vi "PDHydra - TVS Test.vi"(8 "error in (no error)":errorcluster, 10 "Message IN":string) -> (0 "error out":errorcluster, 1 "Result (bool)":bool, 2 "Message OUT":string)   [LabVIEW 2022 SP3]
panel:
  in  "bypass":bool
  in  "stop":bool
  out "Instructional Message":string
  in  "OK Button":bool
  out "Actual Breaker AUX state":bool[](array[boolean])
  out "Result (color)":u32(colorbox)
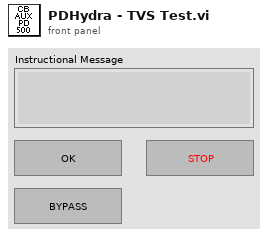
[diagram p1: front panel]
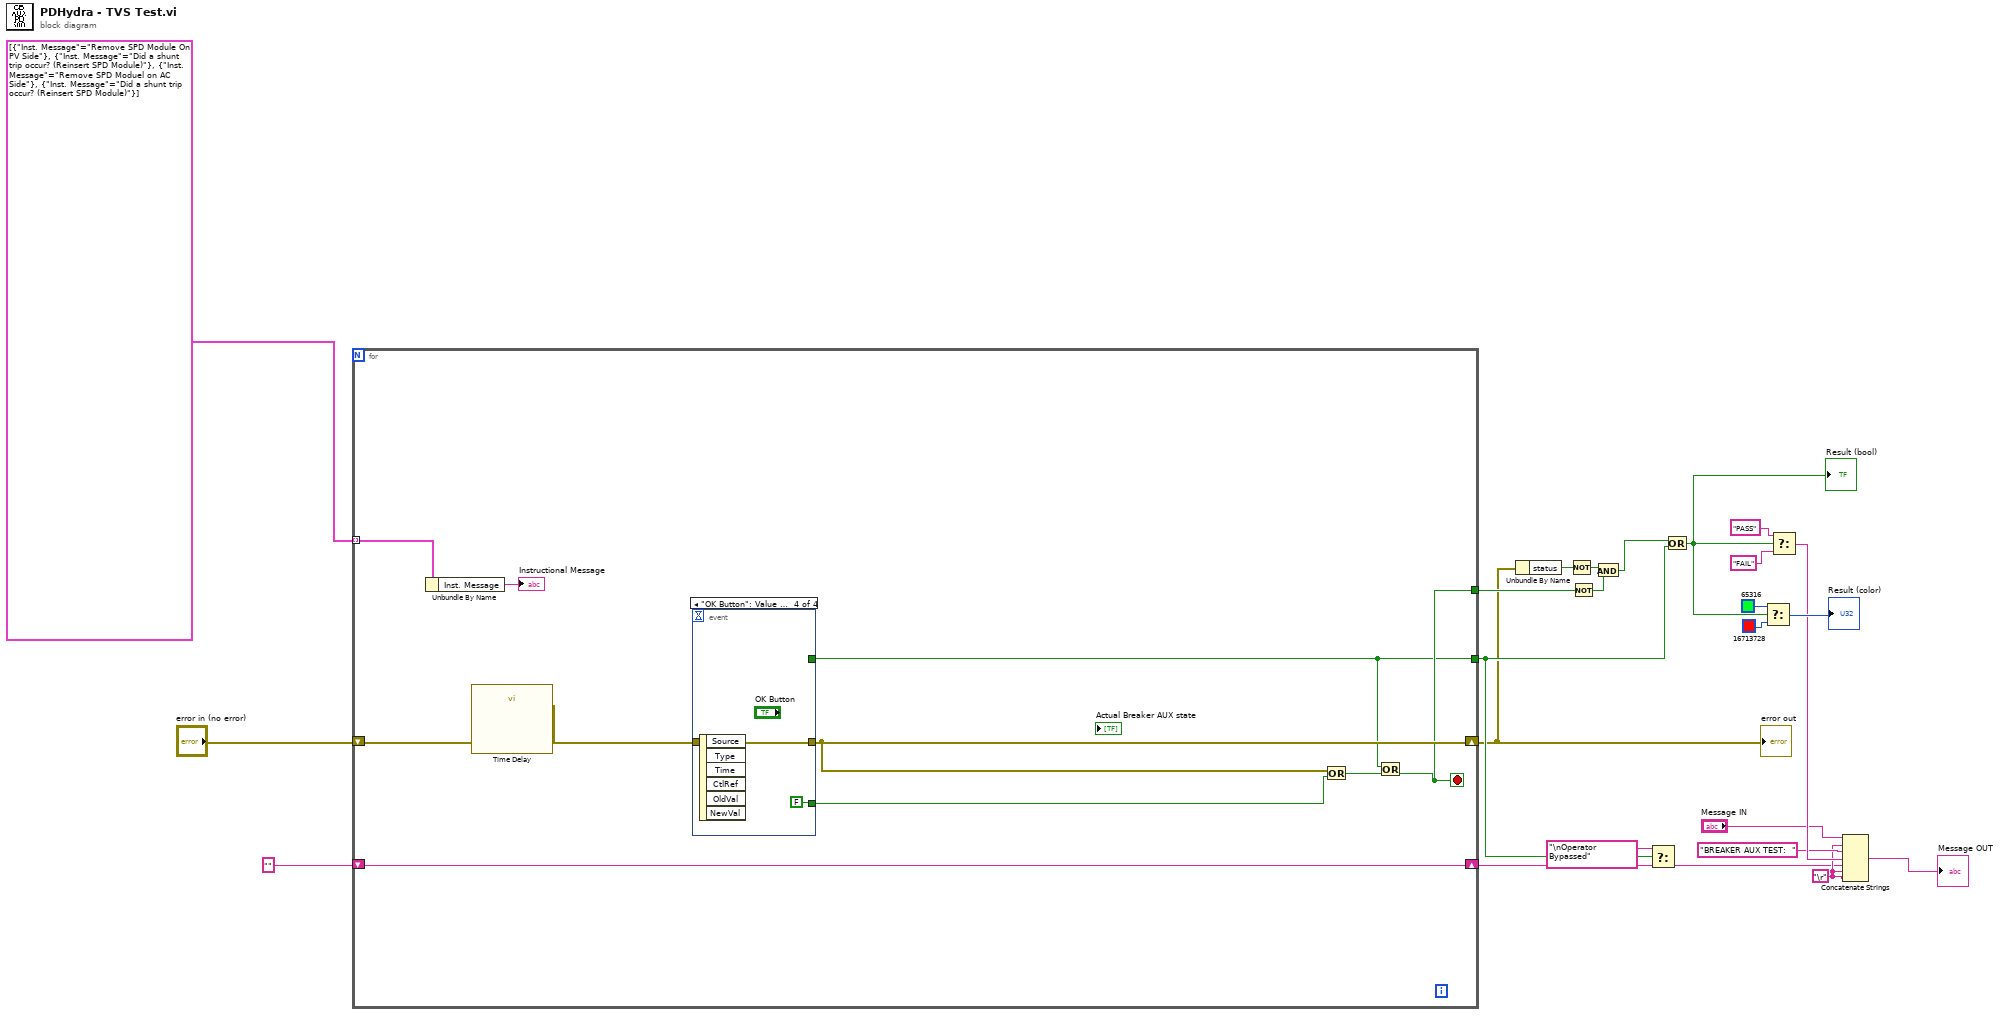
[diagram p0: block diagram]
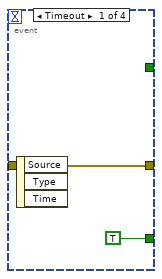
[diagram p2: hidden frame]
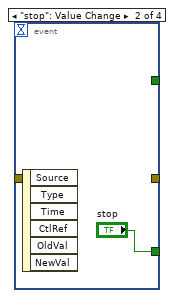
[diagram p3: hidden frame]
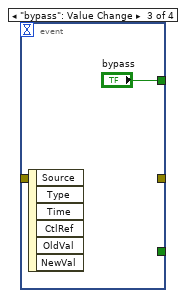
[diagram p4: hidden frame]
diagram:
  w13 = "\r"
  n1 = for {
    shift-right: [w33] -> w1
    shift-left: "error in (no error)" -> [w27]
    shift-right: [w34] -> w4
    shift-left: "" -> [w34]
    tunnel: cluster{"Inst. Message":string}[] [{"Inst. Message"="Remove SPD Module On PV Side"}, {"Inst. Message"="Did a shunt trip occur? (Reinsert SPD Module)"}, {"Inst. Message"="Remove SPD Moduel on AC Side"}, {"Inst. Message"="Did a shunt trip occur? (Reinsert SPD Module)"}] -> [w25] mode=indexing
    tunnel: [w29] -> w8
    tunnel: [w28] -> w3
    stop <- w29 stop-if-true
    n2 = Unbundle By Name(w25) -> ("Inst. Message"=→"Instructional Message":string)
    n3 = call "Time Delay"("error in (no error)"=w27) -> ("error out"=w26:errorcluster)  [unwired: 10 in]
    n4 = event shown="[3] \"OK Button\": Value Change" {
      selector: _ -> [_ _ _ _]
      dyn-events: _ -> [_ _ _ _]
      timeout: _ -> [_ _ _ _]
      tunnel: w26 -> [w36 _ _ w40]
      tunnel: [w36 _ _ w40] -> w33
      tunnel: [TRUE "stop" _ FALSE] -> w31
      tunnel: [_ _ "bypass" _] -> w28
      event Timeout {
        n5 = event-data() -> ()  [unwired: 1 in, 3 out]
      }
      event "stop": Value Change {
        n6 = event-data() -> ()  [unwired: 1 in, 6 out]
      }
      event "bypass": Value Change {
        n7 = event-data() -> ()  [unwired: 1 in, 6 out]
      }
      event "OK Button": Value Change {
        n8 = event-data() -> ()  [unwired: 1 in, 6 out]
      }
    }
    n9 = Or(x=w33, y=w31) -> (x .or. y?=w30:bool)
    n10 = Or(x=w28, y=w30) -> (x .or. y?=w29:bool)
  }
  "error out" <- w1
  n11 = Unbundle By Name(w1) -> ("status"=w19:bool)
  n12 = Not(x=w19) -> (.not. x?=w18:bool)
  n13 = Not(x=w8) -> (.not. x?=w9:bool)
  n14 = And(x=w18, y=w9) -> (x .and. y?=w6:bool)
  n15 = Select(t="\nOperator Bypassed", s=w3, f=w4) -> (s? t:f=w5:string)
  n16 = Or(x=w6, y=w3) -> (x .or. y?=w7:bool)
  "Result (bool)" <- w7
  n17 = Select(t=u32 65316 ("Result (color)"), s=w7, f=u32 16713728 ("Result (color)")) -> (s? t:f=→"Result (color)":u32)
  n18 = Select(t="PASS", s=w7, f="FAIL") -> (s? t:f=w16:string)
  n19 = Concatenate Strings("Message IN", w13, "BREAKER AUX TEST:  ", w16, w5, w13, w13) -> (→"Message OUT":string)
